vi "Calculate Distance.vi"(6 "Robot Calibration Cluster":T1={"Camera Height on robot (in)"=34.5, "Camera Angle on the robot (deg)"=28.3, "Camera FOV Top to Bottom View Angle (deg)"=0.946, "Camera FOV Left to Right View Angle (deg)"=26.5, "Target size (in)"=6.5, "Distance to front of bumper (in)"=10.775, "Focal Length (mm)"=10.0, "Yaw Slope"=12.276, "Yaw Offset"=2.0} {"Yaw Offset" format="%#_13g"; "Yaw Slope" format="%#_13g"; "Camera FOV Left to Right View Angle (deg)" format="%#_13g"; "Focal Length (mm)" format="%#_13g"; "Distance to front of bumper (in)" format="%#_13g"; "Target size (in)" format="%#_13g"; "Camera FOV Top to Bottom View Angle (deg)" format="%#_13g"; "Camera Angle on the robot (deg)" format="%#_13g"; "Camera Height on robot (in)" format="%#_13g"}, 8 "Height to center of target from floor (hp (in))":dbl=98.25 format="%#_13g", 9 "Screen resolution pixels Height (Ry)":dbl=360.0 format="%#_13g", 11 "Middle of target from 0,0 (pixels)":dbl=178.5 format="%#_13g") -> (3 "Distance from target (in)":dbl=116.40675998176638 format="%.2f")   [LabVIEW 2023]
uses:
  April Tags/Camera Info.ctl
panel:
  in  "Camera FOV Top to BottomView Angle (deg)":dbl=49.0 format="%#_13g"
  # "These Items are inputs"
  # "These items should only have to be figured out one time each season unless the camera mounting changes"
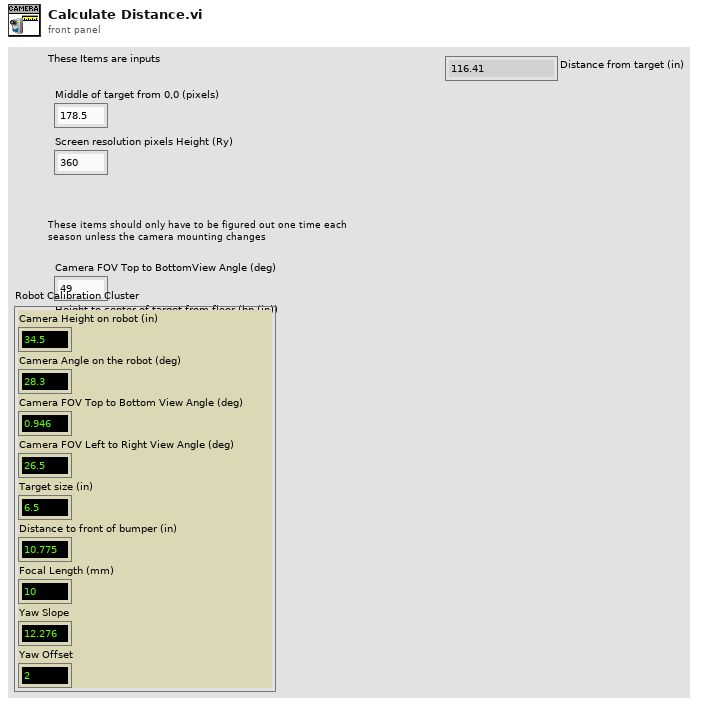
[diagram p1: front panel]
types:
  T1 = typedef "Camera Info.ctl" = cluster{"Camera Height on robot (in)":dbl, "Camera Angle on the robot (deg)":dbl, "Camera FOV Top to Bottom View Angle (deg)":dbl, "Camera FOV Left to Right View Angle (deg)":dbl, "Target size (in)":dbl, "Distance to front of bumper (in)":dbl, "Focal Length (mm)":dbl, "Yaw Slope":dbl, "Yaw Offset":dbl}
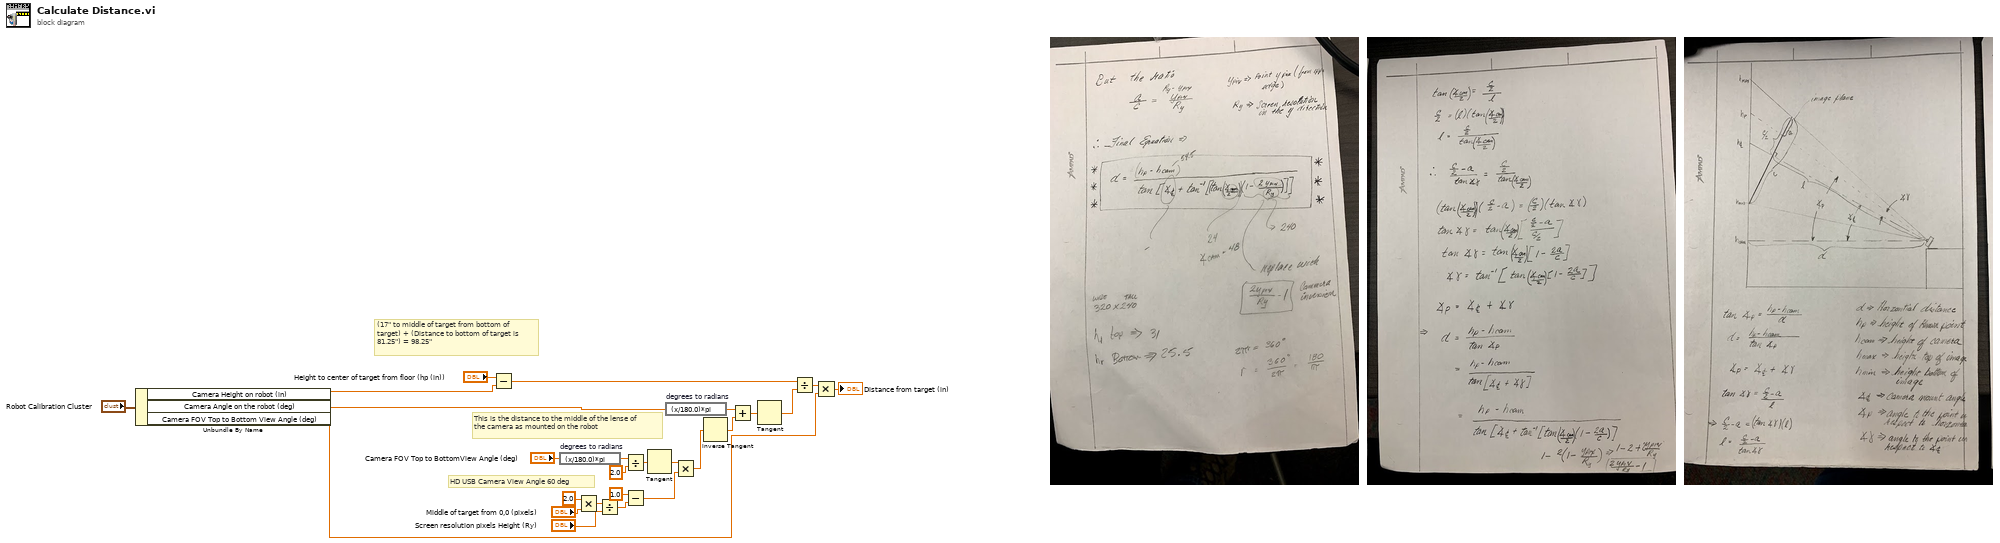
[diagram p0: block diagram]
diagram:
  # "HD USB Camera View Angle 60 deg"
  # "(17\" to middle of target from bottom of target) + (Distance to bottom of target is 81.25\") = 98.25\""
  # "This is the distance to the middle of the lense of the camera as mounted on the robot"
  n1 = Unbundle By Name("Robot Calibration Cluster") -> ("Camera Height on robot (in)"=w4:dbl, "Camera Angle on the robot (deg)"=w3:dbl, "Camera FOV Top to Bottom View Angle (deg)"=w2:dbl)
  n2 = Subtract(x="Height to center of target from floor (hp (in))", y=w4) -> (x-y=w24:dbl)
  n3 = expression code="(x/180.0)*pi" "degrees to radians"("Camera FOV Top to BottomView Angle (deg)") -> (w10:dbl)
  n4 = Multiply(x=2.0, y="Middle of target from 0,0 (pixels)") -> (x*y=w19:dbl)
  n5 = Divide(x=w19, y="Screen resolution pixels Height (Ry)") -> (x/y=w17:dbl)
  n6 = Divide(x=w10, y=2.0) -> (x/y=w15:dbl)
  n7 = Subtract(x=1.0, y=w17) -> (x-y=w13:dbl)
  n8 = Tangent(1:w15) -> (0:w14:dbl)
  n9 = expression code="(x/180.0)*pi" "degrees to radians"(w3) -> (w9:dbl)
  n10 = Multiply(x=w14, y=w13) -> (x*y=w12:dbl)
  n11 = Inverse Tangent(1:w12) -> (0:w23:dbl)
  n12 = Add(x=w9, y=w23) -> (x+y=w8:dbl)
  n13 = Tangent(1:w8) -> (0:w7:dbl)
  n14 = Divide(x=w24, y=w7) -> (x/y=w6:dbl)
  n15 = Multiply(x=w6, y=w2) -> (x*y=→"Distance from target (in)":dbl)
